vi "center.vi"(0 "referenceIn":refnum<k24>, 1 "errorIn":errorcluster, 2 "axis":i32, 3 "travelRange":i32, 4 "averageForwardStepSize":dbl) -> (5 "referenceOut":refnum<k24>, 6 "errorOut":errorcluster)   [LabVIEW 2013]
uses:
  C:/Program Files/Newport/Piezo Motion Control/Newport AG-UC2-UC8 Applet/Samples/LabVIEW 2009/AgilisCmdLib.dll
  Program Files/Newport/Piezo Motion Control/Newport AG-UC2-UC8 Applet/Samples/LabVIEW 2009/AgilisCmdLib.dll
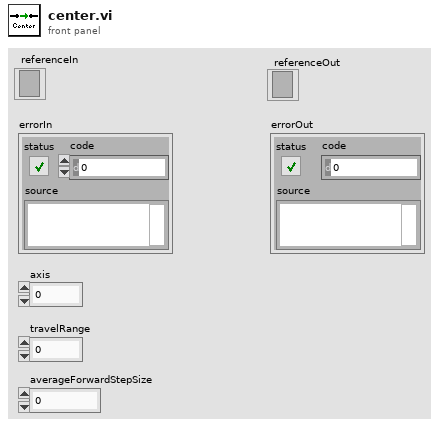
[diagram p1: front panel]
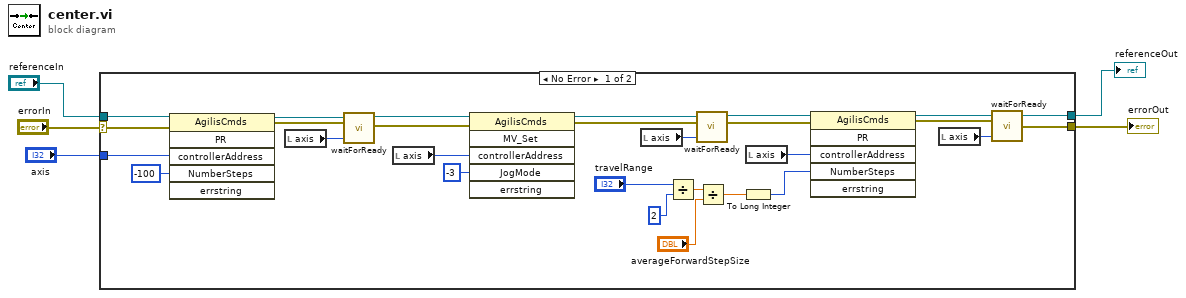
[diagram p0: block diagram]
diagram:
  n1 = case shown="No Error" "errorIn" {
    selector: "errorIn" -> [w15 w35]
    tunnel: "referenceIn" -> [w16 w34]
    tunnel: "axis" -> [w14 _]
    tunnel: [w19 w35] -> w2
    tunnel: [w18 w34] -> w1
    frame No Error {
      n2 = invoke class="AgilisCmds" method="PR"(reference=w16, error in=w15, "controllerAddress"=w14, "NumberSteps"=i64 -100) -> (reference out=w10:refnum<k24>, error out=w8:errorcluster)  [unwired: 2 in, 4 out]
      n3 = local read "axis"() -> (w6:i32)
      n4 = call "waitForReady.vi"("axis"=w6, "errorIn"=w8, "referenceIn"=w10) -> ("errorOut"=w7:errorcluster, "referenceOut"=w9:refnum<k24>)
      n5 = local read "axis"() -> (w12:i32)
      n6 = invoke class="AgilisCmds" method="MV_Set"(reference=w9, error in=w7, "controllerAddress"=w12, "JogMode"=-3) -> (reference out=w33:refnum<k24>, error out=w32:errorcluster)  [unwired: 2 in, 4 out]
      n7 = local read "axis"() -> (w31:i32)
      n8 = Divide(x="travelRange", y=2) -> (x/y=w25:dbl)
      n9 = call "waitForReady.vi"("axis"=w31, "errorIn"=w32, "referenceIn"=w33) -> ("errorOut"=w29:errorcluster, "referenceOut"=w30:refnum<k24>)
      n10 = Divide(x=w25, y="averageForwardStepSize") -> (x/y=w23:dbl)
      n11 = To Long Integer(number=w23) -> (32bit integer=w22:i32)
      n12 = local read "axis"() -> (w28:i32)
      n13 = invoke class="AgilisCmds" method="PR"(reference=w30, error in=w29, "controllerAddress"=w28, "NumberSteps"=w22) -> (reference out=w21:refnum<k24>, error out=w20:errorcluster)  [unwired: 2 in, 4 out]
      n14 = local read "axis"() -> (w17:i32)
      n15 = call "waitForReady.vi"("axis"=w17, "errorIn"=w20, "referenceIn"=w21) -> ("errorOut"=w19:errorcluster, "referenceOut"=w18:refnum<k24>)
    }
    frame Error {
    }
  }
  "referenceOut" <- w1
  "errorOut" <- w2
